vi "Get Path UI.vi"() -> ()   [LabVIEW 2016, in "LV-Data.PGSQL.lvclass"]
uses:
  LV-Data.PGSQL.lvclass
panel:
  out "path_to_selected_column":string="llab_038:d001(TEST_TABLE--new_stuff(hippos))"
  out "selected_table":string="TEST_TABLE"
  in  "columns_list":i32(listbox)=1
  in  "tables_list":i32(listbox)=34
  in  "STOP":bool
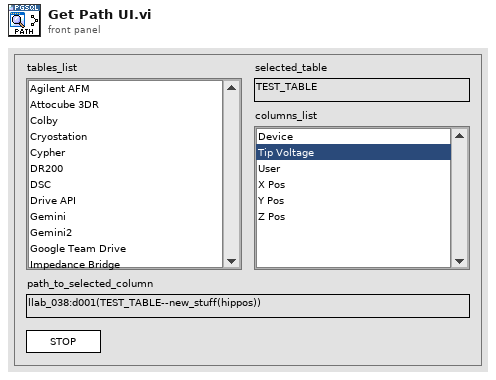
[diagram p1: front panel]
types:
  T1 = enum32{"Invalid", "Standard", "Closed", "Hidden", "Minimized", "Maximized"}
  T2 = enum32{"invalid app kind", "Development System", "Run Time System", "Student Edition", "Embedded LabVIEW", "Evaluation", "Custom"}
  T3 = cluster{"Core":cluster{"Current VI Reference":refnum<vi>, "Close Panel on Exit?":bool}, "Data.PG":refnum<class "LV-Data.PGSQL.lvclass">, "table names":string[], "table paths":string[], "column names":string[], "column units":string[], "column paths":string[], "new table name":string, "new column name":string, "new column data type":string, "new column units":string, "selected table":string, "selected column":string, "selected table path":string, "selected column path":string, "max points":i32, "selected column units":string}
  T4 = cluster{"Current VI Reference":refnum<vi>, "Close Panel on Exit?":bool}
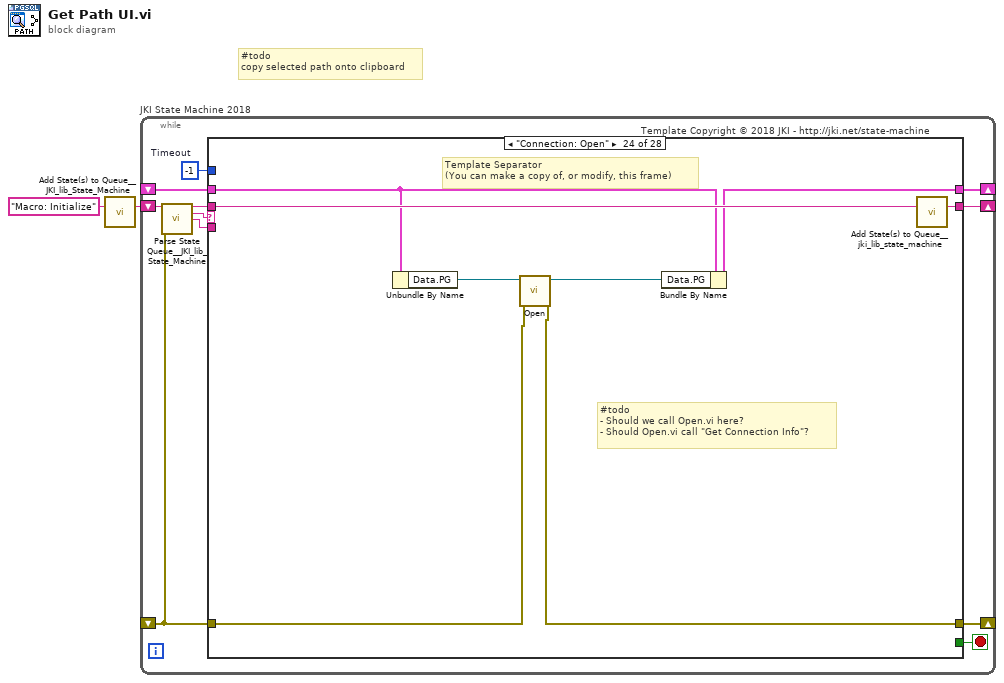
[diagram p0: block diagram]
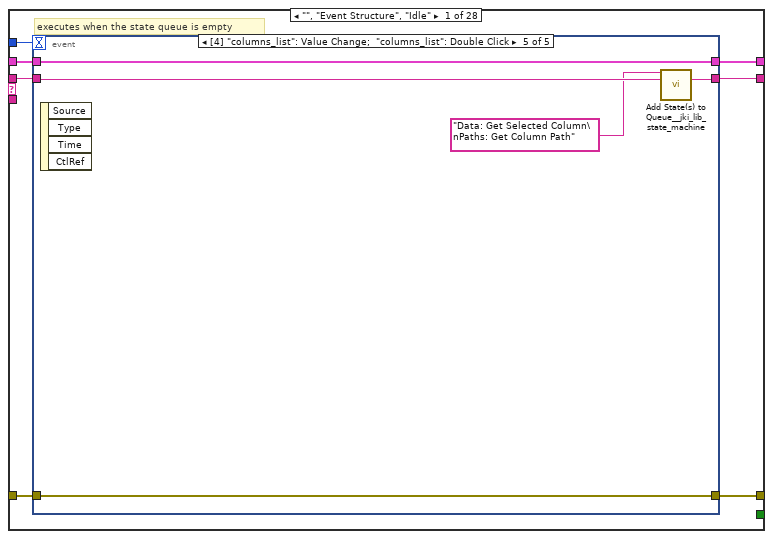
[diagram p2: hidden frame]
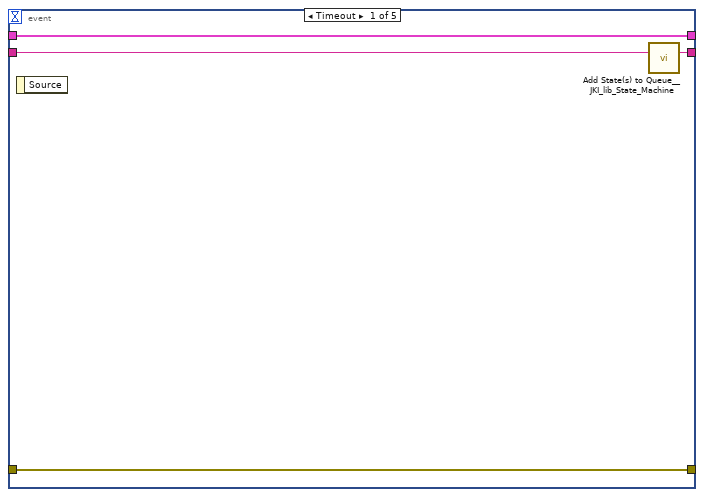
[diagram p3: hidden frame]
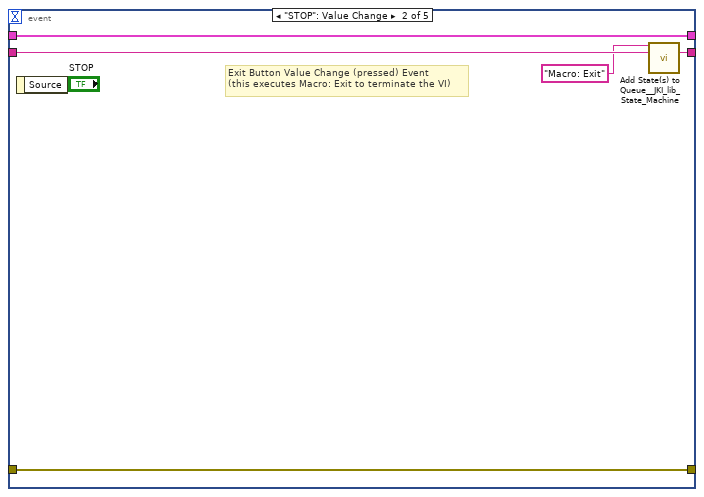
[diagram p4: hidden frame]
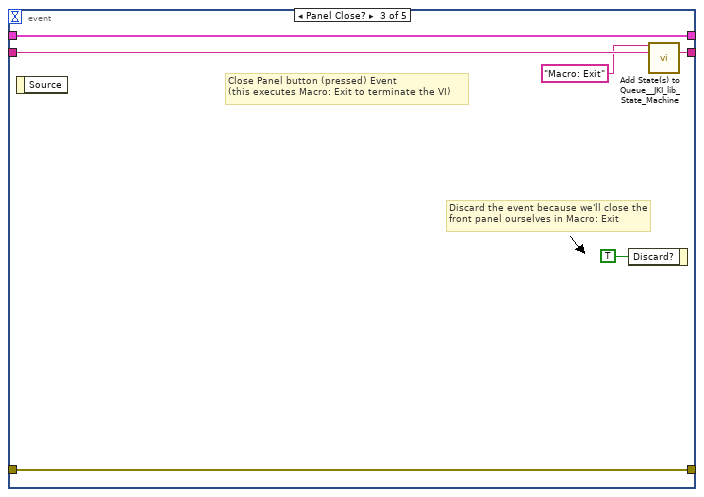
[diagram p5: hidden frame]
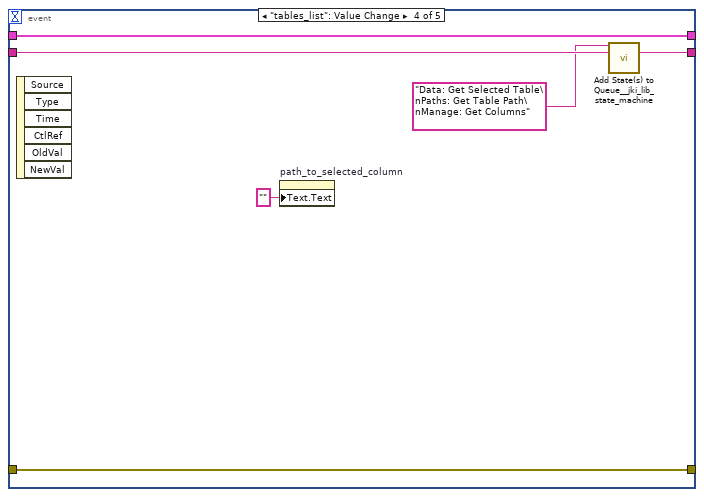
[diagram p6: hidden frame]
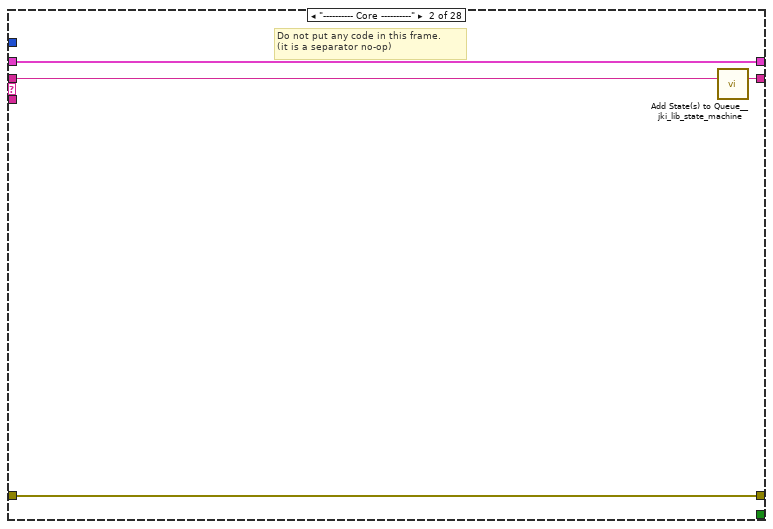
[diagram p7: hidden frame]
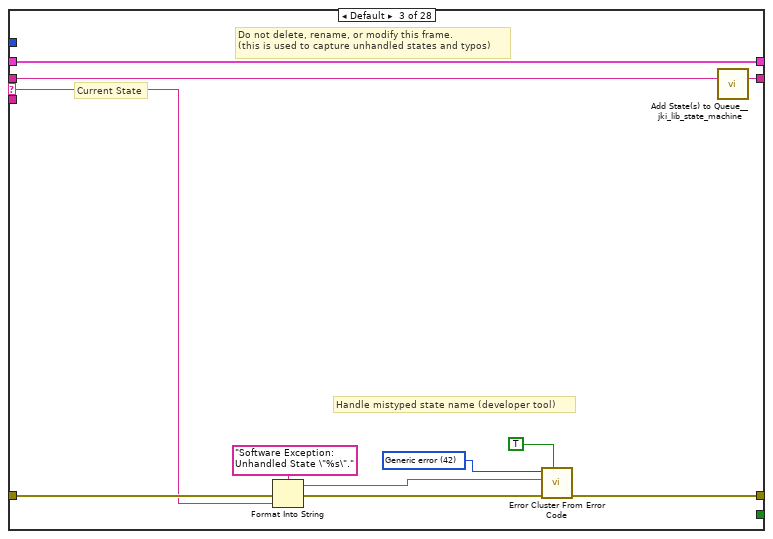
[diagram p8: hidden frame]
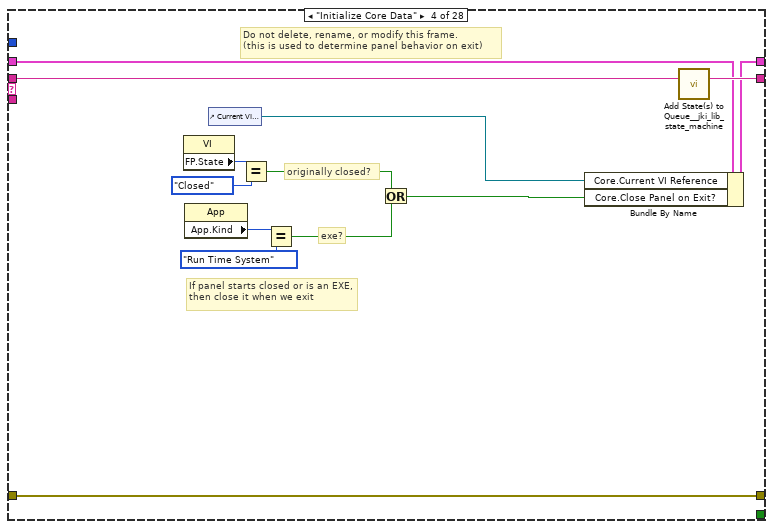
[diagram p9: hidden frame]
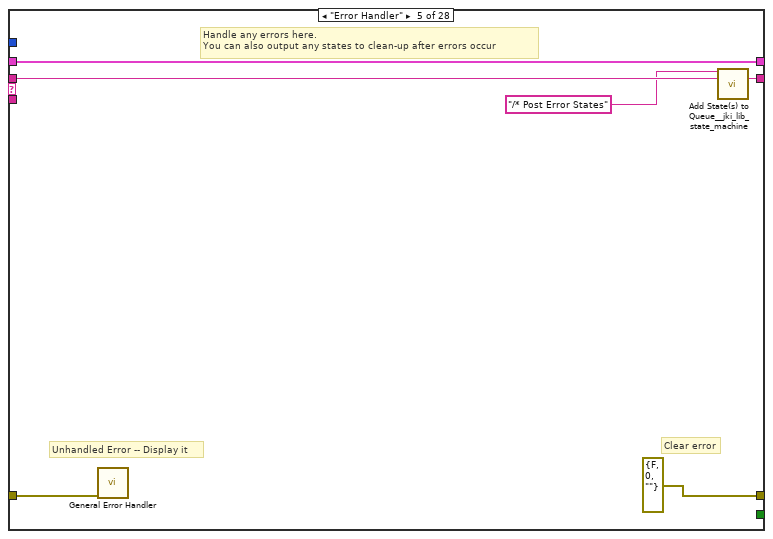
[diagram p10: hidden frame]
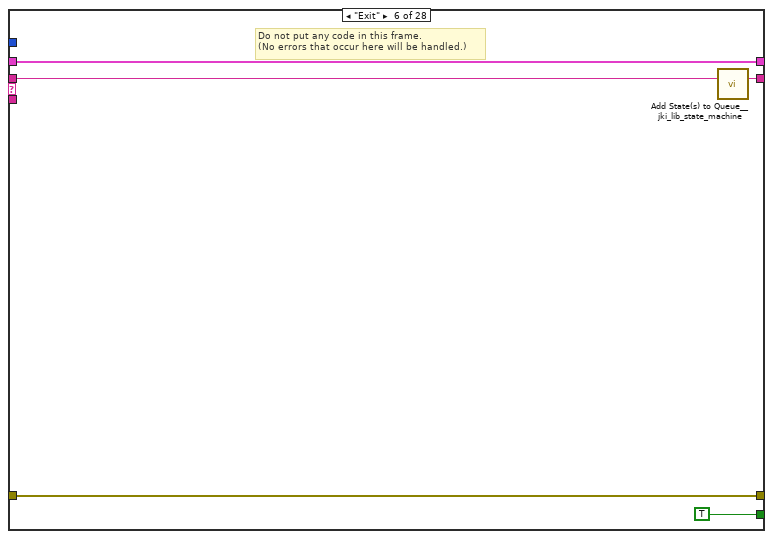
[diagram p11: hidden frame]
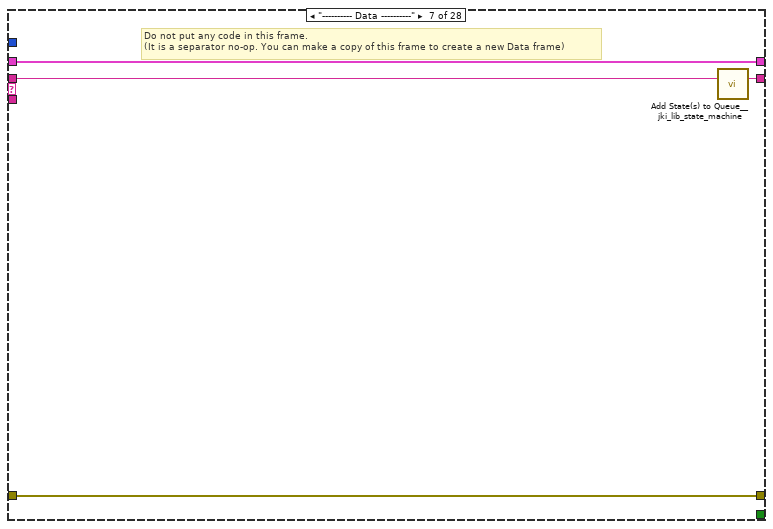
[diagram p12: hidden frame]
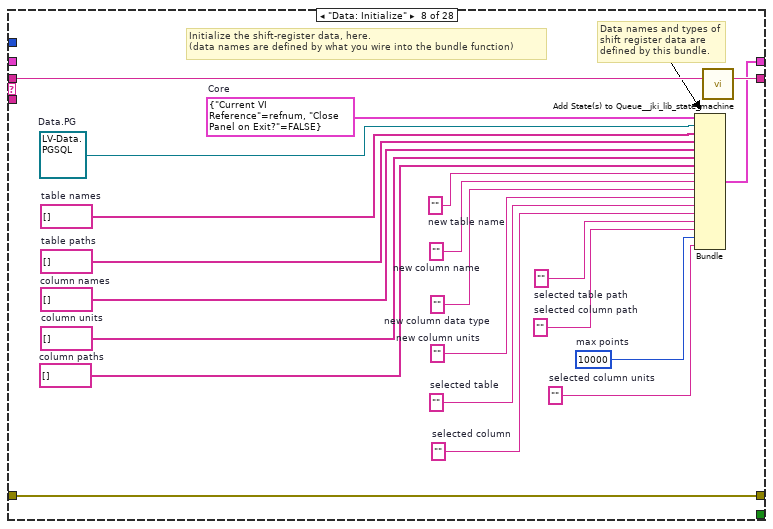
[diagram p13: hidden frame]
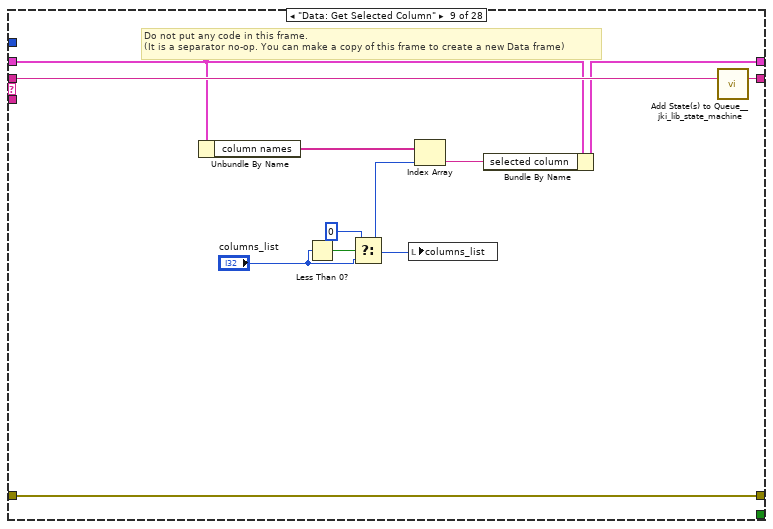
[diagram p14: hidden frame]
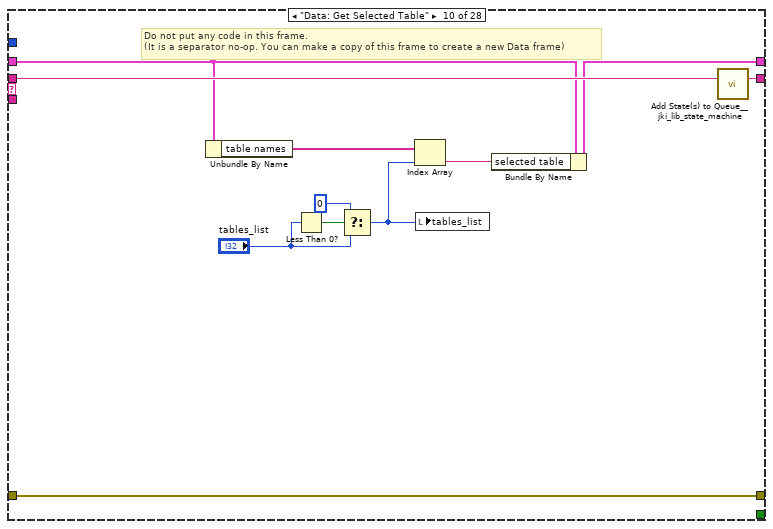
[diagram p15: hidden frame]
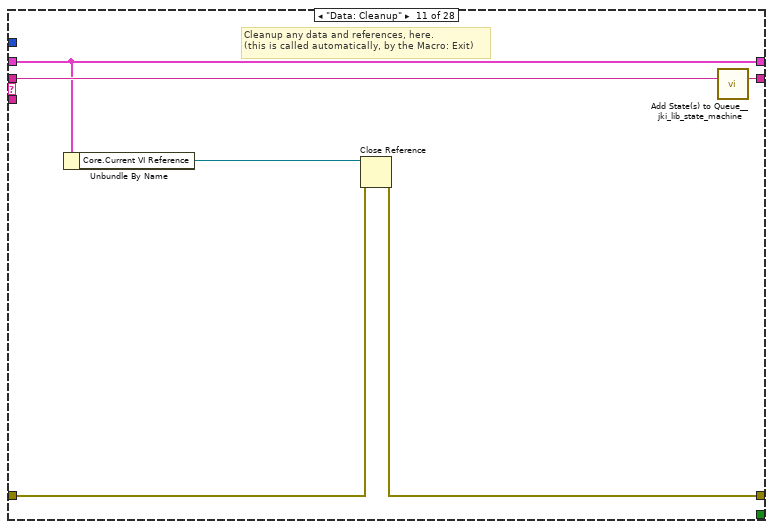
[diagram p16: hidden frame]
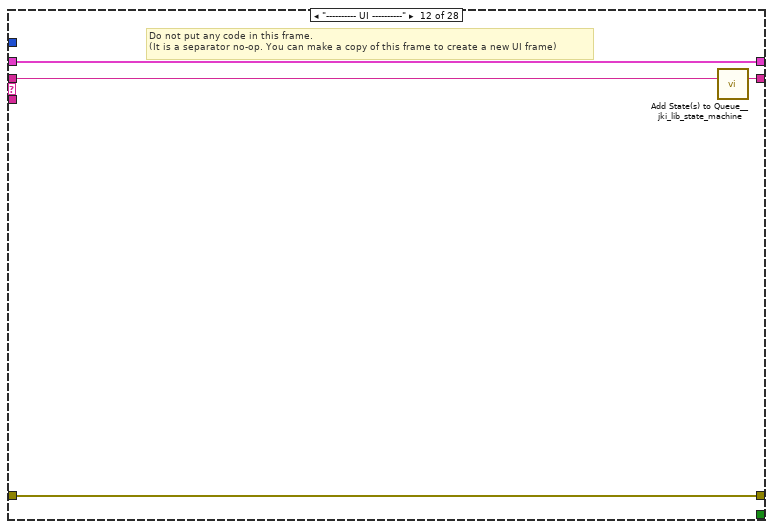
[diagram p17: hidden frame]
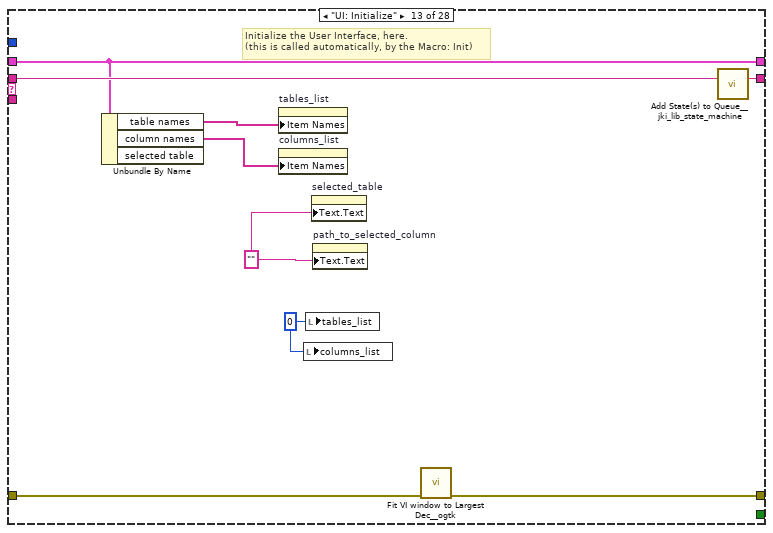
[diagram p18: hidden frame]
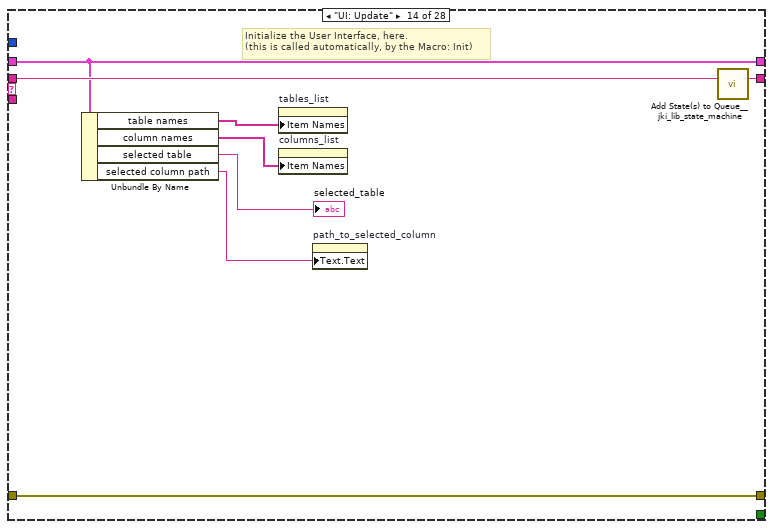
[diagram p19: hidden frame]
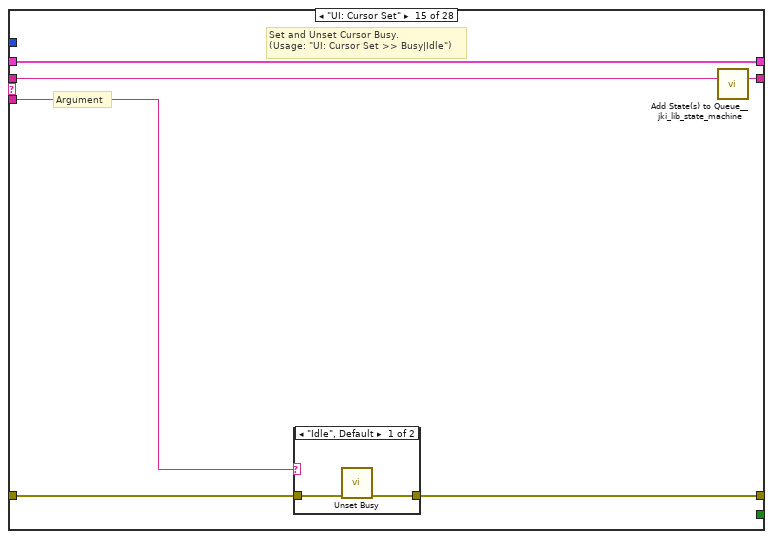
[diagram p20: hidden frame]
diagram:
  # "#todo\ncopy selected path onto clipboard"
  n1 = call <vilib>:"Add State(s) to Queue__JKI_lib_State_Machine.vi"("State(s) in (\"\")"="Macro: Initialize") -> ("States Out"=w2:string)  [unwired: 14 in]
  n2 = while "JKI State Machine 2018" {
    shift-right: [w6] -> _
    shift-left: _ -> [w5]
    shift-right: [w9] -> _
    shift-left: _ -> [w3]
    shift-right: [w8] -> _
    shift-left: w2 -> [w10]
    stop <- w7 stop-if-true
    w4 = -1  # Timeout
    # "Template Copyright © 2018 JKI - http://jki.net/state-machine"
    n3 = call <vilib>:"Parse State Queue__JKI_lib_State_Machine.vi"("State Queue"=w10, "Error In (no error)"=w3) -> ("Remaining States"=w12:string, "Current State"=w13:string, "Arguments"=w11:string)  [unwired: 11 in]
    n4 = case shown="\"Connection: Open\"" w13 {
      selector: w13 -> [_ _ w51 _ _ _ _ _ _ _ _ _ _ _ _ _ _ _ _ _ _ _ _ _ _ _ _ _]
      tunnel: w12 -> [w20 w50 w55 w74 w80 w85 w89 w110 w121 w132 w138 w142 w151 w159 w165 w176 w245 w250 w260 w264 w273 w286 w290 w298 w304 w308 w317 w331]
      tunnel: w11 -> [_ _ _ _ _ _ _ _ _ _ _ _ _ _ w160 w170 _ _ _ _ _ _ _ _ _ _ _ _]
      tunnel: w5 -> [w18 w47 w53 w67 w77 w83 w86 _ w116 w127 w134 w139 w147 w156 w163 w172 w242 w247 w257 w261 w269 w278 w287 w296 w302 w305 w313 w318]
      tunnel: [w17 w48 w57 w71 errorcluster {"status"=FALSE, "code"=0, "source"=""} ("error out") w82 w87 w107 w119 w130 w135 w140 w146 w155 w161 w173 w243 w248 w258 w262 w267 w280 w288 w292 w299 w306 w310 w326] -> w9
      tunnel: w3 -> [w16 w48 w56 w71 w76 w82 w87 w107 w119 w130 w133 w140 w145 w155 w162 w174 w243 w248 w258 w262 w268 w281 w288 w293 w300 w306 w311 w327]
      tunnel: [w19 w49 w54 w73 w79 w84 w88 w109 w120 w131 w137 w141 w150 w158 w164 w175 w244 w249 w259 w263 w272 w285 w289 w297 w303 w307 w316 w330] -> w8
      tunnel: [_ _ _ _ _ TRUE _ _ _ _ _ _ _ _ _ _ _ _ _ _ _ _ _ _ _ _ _ _] -> w7
      tunnel: [w15 w47 w53 w72 w77 w83 w86 w108 w115 w126 w134 w139 w147 w156 w163 w172 w242 w247 w257 w261 w270 w279 w287 w295 w302 w305 w309 w328] -> w6
      tunnel: w4 -> [w14 _ _ _ _ _ _ _ _ _ _ _ _ _ _ _ _ _ _ _ _ _ _ _ _ _ _ _]
      frame "", "Event Structure", "Idle" {
        # "executes when the state queue is empty"
        n5 = event shown="[4] \"columns_list\": Value Change;  \"columns_list\": Double Click" {
          selector: _ -> [_ _ _ _ _]
          dyn-events: _ -> [_ _ _ _ _]
          timeout: w14 -> [_ _ _ _ _]
          tunnel: w20 -> [w24 w29 w35 w39 w45]
          tunnel: [w23 w28 w34 w40 w46] -> w19
          tunnel: w18 -> [w21 w26 w32 w36 w42]
          tunnel: [w22 w27 w33 w41 w43] -> w17
          tunnel: w16 -> [w22 w27 w33 w41 w43]
          tunnel: [w21 w26 w32 w36 w42] -> w15
          event Timeout {
            n6 = event-data() -> ()  [unwired: 1 in, 1 out]
            n7 = call <vilib>:"Add State(s) to Queue__JKI_lib_State_Machine.vi"("State(s) in (\"\")"=w24) -> ("States Out"=w23:string)  [unwired: 14 in]
          }
          event "STOP": Value Change {
            # "Exit Button Value Change (pressed) Event\n(this executes Macro: Exit to terminate the VI)"
            n8 = event-data() -> ()  [unwired: 1 in, 1 out]
            n9 = call <vilib>:"Add State(s) to Queue__JKI_lib_State_Machine.vi"("State(s) in Front (\"\")"="Macro: Exit", "State(s) in (\"\")"=w29) -> ("States Out"=w28:string)  [unwired: 13 in]
          }
          event Panel Close? {
            # "Discard the event because we'll close the front panel ourselves in Macro: Exit"
            # "Close Panel button (pressed) Event\n(this executes Macro: Exit to terminate the VI)"
            n10 = event-data() -> ()  [unwired: 1 in, 1 out]
            n11 = event-data("Discard?"=TRUE) -> ()  [unwired: 1 in, 1 out]
            n12 = call <vilib>:"Add State(s) to Queue__JKI_lib_State_Machine.vi"("State(s) in Front (\"\")"="Macro: Exit", "State(s) in (\"\")"=w35) -> ("States Out"=w34:string)  [unwired: 13 in]
          }
          event "tables_list": Value Change {
            n13 = event-data() -> ()  [unwired: 1 in, 6 out]
            n14 = property on="path_to_selected_column" class="Str"("Text.Text"="") -> ()  [unwired: 2 in, 2 out]
            n15 = call <vilib>:"Add State(s) to Queue__jki_lib_state_machine.vi"("State(s) in Front (\"\")"="Data: Get Selected Table\nPaths: Get Table Path\nManage: Get Columns" ("State(s) in Front (\"\")"), "State(s) in (\"\")"=w39) -> ("States Out"=w40:string)  [unwired: 13 in]
          }
          event "columns_list": Value Change; "columns_list": Double Click {
            n16 = event-data() -> ()  [unwired: 1 in, 4 out]
            n17 = call <vilib>:"Add State(s) to Queue__jki_lib_state_machine.vi"("State(s) in Front (\"\")"="Data: Get Selected Column\nPaths: Get Column Path", "State(s) in (\"\")"=w45) -> ("States Out"=w46:string)  [unwired: 13 in]
          }
        }
      }
      frame "---------- Core ----------" {
        # "Do not put any code in this frame.\n(it is a separator no-op)"
        n18 = call <vilib>:"Add State(s) to Queue__jki_lib_state_machine.vi"("State(s) in (\"\")"=w50) -> ("States Out"=w49:string)  [unwired: 14 in]
      }
      frame Default {
        w60 = 42 items=["No error", "Argument error", "Memory is full", "Out of zone", "End of file", "File already open", "Generic file I/O error", "File not found", "File permission error", "Disk is full", "Duplicate path", "Too many files open", "System feature not enabled", "Resource file not found", "Cannot add resource", "Resource not found", "Image not found", "Image memory error", "Pen does not exist", "Config type invalid", "Config token not found", "Config parse error", "Config memory error", "Bad external code format", "Bad external code offset", "External code not present", "Null window", "Destroy window error", "Null menu", "Print aborted", "Bad print record", "Print driver error", "Windows error during printing", "Memory error during printing", "Print dialog error", "Generic print error", "Invalid device refnum", "Device not found", "Device parameter error", "Device unit error", "Cannot open device", "Device call aborted", "Generic error", "Cancelled by user", "Object ID too low", "Object ID too high", "Object not in heap", "Unknown heap", "Unknown object (invalid DefProc)", "Unknown object (DefProc not in table)", "Message out of range", "Invalid (null) method", "Unknown message", "Manager call not supported", "Bad address", "Network operation in progress", "Network operation timed out", "Connection is busy", "Network attribute not supported", "Network error", "Address in use", "System out of memory", "Connection aborted", "Connection refused", "Not connected", "Already connected", "Connection closed", "Initialization error (interapplication manager)", "Bad occurrence", "Wait on unbound occurrence handler", "Occurrence queue overflow", "Datalog type conflict", "Unused", "Unrecognized type (interapplication manager)", "Memory corrupt", "Failed to make temporary DLL", "Old CIN version", "Drag socket not found", "Failed to load drop-object", "Failed to register OLE object", "Failed to release OLE object", "Format specifier type mismatch", "Unknown format specifier", "Too few format specifiers", "Too many format specifiers", "Scan failed", "Newer CIN version", "Error converting to variant", "Runtime menu error", "Password tampered", "Variant attribute not found", "Incompatible variant data type", "Event data is not available", "Event Store is not present", "Occurrence is not found", "Event Queue is not created", "Event info is not available", "Refnum passed is NULL", "Error retrieving Class GUID", "Error retrieving CoClass GUID", "Error retrieving TypeLib GUID.", "Bad built application magic bytes.", "Specific driver is different from the specific driver associated with the Logical Name.", "There is no session opened to the class driver.", "Max Error", "MAX - Error with config objects", "MAX - Error loading configuration", "MAX - Group not supported"]
        # "Current State"
        # "Do not delete, rename, or modify this frame.\n(this is used to capture unhandled states and typos)"
        # "Handle mistyped state name (developer tool)"
        n19 = Format Into String(format string="Software Exception: Unhandled State \"%s\"." ("message"), error in=w56, w51) -> (resulting string=w59:string, error out=w58:errorcluster)  [unwired: 1 in]
        n20 = call <vilib>:"Error Cluster From Error Code.vi"("show call chain? (False)"=TRUE, "error in (no error)"=w58, "error message (\"\")"=w59, "error code (0)"=w60) -> ("error out"=w57:errorcluster)  [unwired: 5 in]
        n21 = call <vilib>:"Add State(s) to Queue__jki_lib_state_machine.vi"("State(s) in (\"\")"=w55) -> ("States Out"=w54:string)  [unwired: 14 in]
      }
      frame "Initialize Core Data" {
        # "Do not delete, rename, or modify this frame.\n(this is used to determine panel behavior on exit)"
        # "originally closed?"
        # "exe?"
        # "If panel starts closed or is an EXE, then close it when we exit"
        n22 = property class="VI"() -> ("FP.State"=w64:T1)  [unwired: 2 in, 2 out]
        n23 = property class="App"() -> ("App.Kind"=w70:T2)  [unwired: 2 in, 2 out]
        n24 = control-ref of="Current VI Reference"() -> (w65:refnum<vi>)
        n25 = Equal?(x=w64, y=T1."Closed" ("Front Panel Window:State")) -> (x = y?=w62:bool)
        n26 = Equal?(x=w70, y=T2."Run Time System" ("Application:Kind")) -> (x = y?=w68:bool)
        n27 = Or(x=w62, y=w68) -> (x .or. y?=w66:bool)
        n28 = Bundle By Name(cluster=w67, "Core.Current VI Reference"=w65, "Core.Close Panel on Exit?"=w66) -> (w72:T3)
        n29 = call <vilib>:"Add State(s) to Queue__jki_lib_state_machine.vi"("State(s) in (\"\")"=w74) -> ("States Out"=w73:string)  [unwired: 14 in]
      }
      frame "Error Handler" {
        # "Unhandled Error -- Display it"
        # "Handle any errors here.\nYou can also output any states to clean-up after errors occur"
        # "Clear error"
        n30 = call <vilib>:"General Error Handler.vi"("error in (no error)"=w76) -> ()  [unwired: 10 in, 5 out]
        n31 = call <vilib>:"Add State(s) to Queue__jki_lib_state_machine.vi"("State(s) in Front (\"\")"="/* Post Error States", "State(s) in (\"\")"=w80) -> ("States Out"=w79:string)  [unwired: 13 in]
      }
      frame "Exit" {
        # "Do not put any code in this frame.\n(No errors that occur here will be handled.)"
        n32 = call <vilib>:"Add State(s) to Queue__jki_lib_state_machine.vi"("State(s) in (\"\")"=w85) -> ("States Out"=w84:string)  [unwired: 14 in]
      }
      frame "---------- Data ----------" {
        # "Do not put any code in this frame.\n(It is a separator no-op. You can make a copy of this frame to create a new Data frame)"
        n33 = call <vilib>:"Add State(s) to Queue__jki_lib_state_machine.vi"("State(s) in (\"\")"=w89) -> ("States Out"=w88:string)  [unwired: 14 in]
      }
      frame "Data: Initialize" {
        w90 = ""  # selected column units
        w91 = 10000  # max points
        w92 = ""  # selected column path
        w93 = ""  # selected table path
        w94 = ""  # selected column
        w95 = ""  # selected table
        w96 = ""  # new column units
        w97 = ""  # new column data type
        w98 = ""  # new column name
        w99 = ""  # new table name
        w100 = string[] []  # column paths
        w101 = string[] []  # column units
        w102 = string[] []  # column names
        w103 = string[] []  # table paths
        w104 = string[] []  # table names
        w105 = refnum<class "LV-Data.PGSQL.lvclass"> refnum  # Data.PG
        w106 = T4 {"Current VI Reference"=refnum, "Close Panel on Exit?"=FALSE}  # Core
        # "Data names and types of shift register data are defined by this bundle."
        # "Initialize the shift-register data, here.\n(data names are defined by what you wire into the bundle function)"
        n34 = Bundle("Core"=w106, "Data.PG"=w105, "table names"=w104, "table paths"=w103, "column names"=w102, "column units"=w101, "column paths"=w100, "new table name"=w99, "new column name"=w98, "new column data type"=w97, "new column units"=w96, "selected table"=w95, "selected column"=w94, "selected table path"=w93, "selected column path"=w92, "max points"=w91, "selected column units"=w90) -> (w108:T3)  [unwired: 1 in]
        n35 = call <vilib>:"Add State(s) to Queue__jki_lib_state_machine.vi"("State(s) in (\"\")"=w110) -> ("States Out"=w109:string)  [unwired: 14 in]
      }
      frame "Data: Get Selected Column" {
        # "Do not put any code in this frame.\n(It is a separator no-op. You can make a copy of this frame to create a new Data frame)"
        n36 = Unbundle By Name(w116) -> ("column names"=w118:string[])
        n37 = Less Than 0?(x="columns_list") -> (x < 0?=w114:bool)
        n38 = Select(t=0, s=w114, f="columns_list") -> (s? t:f=w111:i32)
        n39 = local write "columns_list"(w111) -> ()
        n40 = Index Array(array=w118, index=w111) -> (element=w117:string)
        n41 = Bundle By Name(cluster=w116, "selected column"=w117) -> (w115:T3)
        n42 = call <vilib>:"Add State(s) to Queue__jki_lib_state_machine.vi"("State(s) in (\"\")"=w121) -> ("States Out"=w120:string)  [unwired: 14 in]
      }
      frame "Data: Get Selected Table" {
        # "Do not put any code in this frame.\n(It is a separator no-op. You can make a copy of this frame to create a new Data frame)"
        n43 = Unbundle By Name(w127) -> ("table names"=w129:string[])
        n44 = Less Than 0?(x="tables_list") -> (x < 0?=w125:bool)
        n45 = Select(t=0, s=w125, f="tables_list") -> (s? t:f=w123:i32)
        n46 = Index Array(array=w129, index=w123) -> (element=w128:string)
        n47 = local write "tables_list"(w123) -> ()
        n48 = Bundle By Name(cluster=w127, "selected table"=w128) -> (w126:T3)
        n49 = call <vilib>:"Add State(s) to Queue__jki_lib_state_machine.vi"("State(s) in (\"\")"=w132) -> ("States Out"=w131:string)  [unwired: 14 in]
      }
      frame "Data: Cleanup" {
        # "Cleanup any data and references, here.\n(this is called automatically, by the Macro: Exit)"
        n50 = Unbundle By Name(w134) -> ("Core.Current VI Reference"=w136:refnum<vi>)
        n51 = Close Reference(reference=w136, error in (no error)=w133) -> (error out=w135:errorcluster)
        n52 = call <vilib>:"Add State(s) to Queue__jki_lib_state_machine.vi"("State(s) in (\"\")"=w138) -> ("States Out"=w137:string)  [unwired: 14 in]
      }
      frame "---------- UI ----------" {
        # "Do not put any code in this frame.\n(It is a separator no-op. You can make a copy of this frame to create a new UI frame)"
        n53 = call <vilib>:"Add State(s) to Queue__jki_lib_state_machine.vi"("State(s) in (\"\")"=w142) -> ("States Out"=w141:string)  [unwired: 14 in]
      }
      frame "UI: Initialize" {
        w144 = 0 ("tables_list")
        w143 = "" ("Text.Text")
        # "Initialize the User Interface, here.\n(this is called automatically, by the Macro: Init)"
        n54 = Unbundle By Name(w147) -> ("table names"=w149:string[], "column names"=w148:string[])  [unwired: 1 out]
        n55 = property on="tables_list" class="LstBox (strict)"("Item Names"=w149) -> ()  [unwired: 2 in, 2 out]
        n56 = property on="columns_list" class="LstBox (strict)"("Item Names"=w148) -> ()  [unwired: 2 in, 2 out]
        n57 = local write "columns_list"(w144) -> ()
        n58 = local write "tables_list"(w144) -> ()
        n59 = property on="selected_table" class="Str"("Text.Text"=w143) -> ()  [unwired: 2 in, 2 out]
        n60 = property on="path_to_selected_column" class="Str"("Text.Text"=w143) -> ()  [unwired: 2 in, 2 out]
        n61 = call <userlib>:"Fit VI window to Largest Dec__ogtk.vi"("error in (no error)"=w145) -> ("error out"=w146:errorcluster)  [unwired: 5 in, 1 out]
        n62 = call <vilib>:"Add State(s) to Queue__jki_lib_state_machine.vi"("State(s) in (\"\")"=w151) -> ("States Out"=w150:string)  [unwired: 14 in]
      }
      frame "UI: Update" {
        # "Initialize the User Interface, here.\n(this is called automatically, by the Macro: Init)"
        n63 = Unbundle By Name(w156) -> ("table names"=w157:string[], "column names"=w153:string[], "selected table"=→"selected_table":string, "selected column path"=w152:string)
        n64 = property on="tables_list" class="LstBox (strict)"("Item Names"=w157) -> ()  [unwired: 2 in, 2 out]
        n65 = property on="columns_list" class="LstBox (strict)"("Item Names"=w153) -> ()  [unwired: 2 in, 2 out]
        n66 = property on="path_to_selected_column" class="Str"("Text.Text"=w152) -> ()  [unwired: 2 in, 2 out]
        n67 = call <vilib>:"Add State(s) to Queue__jki_lib_state_machine.vi"("State(s) in (\"\")"=w159) -> ("States Out"=w158:string)  [unwired: 14 in]
      }
      frame "UI: Cursor Set" {
        # "Argument"
        # "Set and Unset Cursor Busy.\n(Usage: \"UI: Cursor Set >> Busy|Idle\")"
        n68 = case shown="\"Idle\", Default" w160 {
          tunnel: w162 -> [w167 w169]
          tunnel: [w166 w168] -> w161
          frame "Idle", Default {
            n69 = call <vilib>:"Unset Busy.vi"("error in (no error)"=w167) -> ("error out"=w166:errorcluster)  [unwired: 10 in]
          }
          frame "Busy" {
            n70 = call <vilib>:"Set Busy.vi"("error in (no error)"=w169) -> ("error out"=w168:errorcluster)  [unwired: 9 in, 1 out]
          }
        }
        n71 = call <vilib>:"Add State(s) to Queue__jki_lib_state_machine.vi"("State(s) in (\"\")"=w165) -> ("States Out"=w164:string)  [unwired: 14 in]
      }
      frame "UI: Front Panel State" {
        # "Argument"
        # "Set Front Panel Open or Closed\n(Usage: \"UI: Front Panel State >> Open|Close\")"
        n72 = Unbundle By Name(w172) -> ("Core.Current VI Reference"=w171:refnum<vi>)
        n73 = case shown="\"Open\", \"Standard\", Default" w170 {
          tunnel: w174 -> [w182 w197 w208 w221 w234]
          tunnel: [w184 w198 w210 w223 w236] -> w173
          tunnel: w171 -> [w183 w195 w209 w222 w235]
          frame "Open", "Standard", Default {
            w177 = T1."Standard" ("State")
            n74 = property class="VI"(reference=w183, error in=w182) -> (reference out=w180:refnum<vi>, error out=w181:errorcluster, "FP.State"=w179:T1)
            n75 = Not Equal?(x=w179, y=w177) -> (x != y?=w178:bool)
            n76 = case shown="False" w178 {
              tunnel: [w188 w190] -> w184
              tunnel: w181 -> [w187 w190]
              tunnel: w180 -> [w186 _]
              tunnel: w177 -> [w185 _]
              frame True {
                n77 = invoke class="VI" method="FP.Open"(reference=w186, error in=w187, "Activate"=TRUE, "State"=w185) -> (error out=w188:errorcluster)  [unwired: 1 in, 4 out]
              }
              frame False {
              }
            }
          }
          frame "Close", "Closed" {
            n78 = property class="VI"(reference=w195, error in=w197) -> (reference out=w194:refnum<vi>, error out=w196:errorcluster, "FP.State"=w192:T1)
            n79 = Not Equal?(x=w192, y=T1."Closed" ("Front Panel Window:State")) -> (x != y?=w191:bool)
            n80 = case shown="True" w191 {
              tunnel: [w199 w202] -> w198
              tunnel: w196 -> [w199 w201]
              tunnel: w194 -> [_ w200]
              frame False {
              }
              frame True {
                n81 = invoke class="VI" method="FP.Close"(reference=w200, error in=w201) -> (error out=w202:errorcluster)  [unwired: 1 in, 2 out]
              }
            }
          }
          frame "Hidden", "Hide" {
            w203 = T1."Hidden" ("State")
            n82 = property class="VI"(reference=w209, error in=w208) -> (reference out=w206:refnum<vi>, error out=w207:errorcluster, "FP.State"=w205:T1)
            n83 = Not Equal?(x=w205, y=w203) -> (x != y?=w204:bool)
            n84 = case shown="True" w204 {
              tunnel: [w214 w215] -> w210
              tunnel: w207 -> [w213 w215]
              tunnel: w206 -> [w212 _]
              tunnel: w203 -> [w211 _]
              frame True {
                n85 = invoke class="VI" method="FP.Open"(reference=w212, error in=w213, "State"=w211) -> (error out=w214:errorcluster)  [unwired: 2 in, 4 out]
              }
              frame False {
              }
            }
          }
          frame "Minimize", "Minimized" {
            w216 = T1."Minimized" ("State")
            n86 = property class="VI"(reference=w222, error in=w221) -> (reference out=w219:refnum<vi>, error out=w220:errorcluster, "FP.State"=w218:T1)
            n87 = Not Equal?(x=w218, y=w216) -> (x != y?=w217:bool)
            n88 = case shown="True" w217 {
              tunnel: [w227 w228] -> w223
              tunnel: w220 -> [w226 w228]
              tunnel: w219 -> [w225 _]
              tunnel: w216 -> [w224 _]
              frame True {
                n89 = invoke class="VI" method="FP.Open"(reference=w225, error in=w226, "State"=w224) -> (error out=w227:errorcluster)  [unwired: 2 in, 4 out]
              }
              frame False {
              }
            }
          }
          frame "Maximize", "Maximized" {
            w229 = T1."Maximized" ("State")
            n90 = property class="VI"(reference=w235, error in=w234) -> (reference out=w232:refnum<vi>, error out=w233:errorcluster, "FP.State"=w231:T1)
            n91 = Not Equal?(x=w231, y=w229) -> (x != y?=w230:bool)
            n92 = case shown="True" w230 {
              tunnel: [w240 w241] -> w236
              tunnel: w233 -> [w239 w241]
              tunnel: w232 -> [w238 _]
              tunnel: w229 -> [w237 _]
              frame True {
                n93 = invoke class="VI" method="FP.Open"(reference=w238, error in=w239, "State"=w237) -> (error out=w240:errorcluster)  [unwired: 2 in, 4 out]
              }
              frame False {
              }
            }
          }
        }
        n94 = call <vilib>:"Add State(s) to Queue__jki_lib_state_machine.vi"("State(s) in (\"\")"=w176) -> ("States Out"=w175:string)  [unwired: 14 in]
      }
      frame "---------- Macro ----------" {
        # "Do not put any code in this frame.\n(It is a separator no-op. You can make a copy of this frame to create a new Macro frame)"
        n95 = call <vilib>:"Add State(s) to Queue__jki_lib_state_machine.vi"("State(s) in (\"\")"=w245) -> ("States Out"=w244:string)  [unwired: 14 in]
      }
      frame "Macro: Initialize" {
        # "Initialization Macro\n(This is called once, when the VI starts)"
        n96 = call <vilib>:"Add State(s) to Queue__jki_lib_state_machine.vi"("State(s) in Front (\"\")"="Data: Initialize\nInitialize Core Data\nUI: Initialize\nUI: Front Panel State >> Open\n\nConnection: Open\nManage: Get Tables\nUI: Update\n\nData: Get Selected Table\nPaths: Get Table Path\n\nManage: Get Columns\nUI: Update\nData: Get Selected Column\n\nPaths: Get Column Path", "State(s) in (\"\")"=w250) -> ("States Out"=w249:string)  [unwired: 13 in]
      }
      frame "Macro: Exit" {
        # "Exit Macro\n(This is called once, when the VI exits)"
        n97 = Unbundle By Name(w257) -> ("Core.Close Panel on Exit?"=w256:bool)
        n98 = Select(t="UI: Front Panel State >> Close", s=w256, f="") -> (s? t:f=w253:string)
        n99 = call <vilib>:"Add State(s) to Queue__jki_lib_state_machine.vi"("State(s) in (\"\")"=w253, "State(s) at Back (\"\")"="Connection: Close\nData: Cleanup\nExit") -> ("States Out"=w251:string)  [unwired: 13 in]
        n100 = call <vilib>:"Add State(s) to Queue__jki_lib_state_machine.vi"("State(s) in Front (\"\")"=w251, "State(s) in (\"\")"=w260) -> ("States Out"=w259:string)  [unwired: 13 in]
      }
      frame "---------- Manage ----------" {
        # "Template Separator\n(You can make a copy of, or modify, this frame)"
        n101 = call <vilib>:"Add State(s) to Queue__jki_lib_state_machine.vi"("State(s) in (\"\")"=w264) -> ("States Out"=w263:string)  [unwired: 14 in]
      }
      frame "Manage: Get Tables" {
        # "Your code here.\n(You can make a copy of, or modify, this frame)"
        n102 = Unbundle By Name(w269) -> ("Data.PG"=w271:refnum<class "LV-Data.PGSQL.lvclass">)
        n103 = call "Get Tables.vi"("error in (no error)"=w268, "Data.PG"=w271) -> ("error out"=w267:errorcluster, "Table Paths"=w265:string[], "Table Names"=w266:string[])  [unwired: 6 in, 1 out]
        n104 = Bundle By Name(cluster=w269, "table names"=w266, "table paths"=w265) -> (w270:T3)
        n105 = call <vilib>:"Add State(s) to Queue__jki_lib_state_machine.vi"("State(s) in (\"\")"=w273) -> ("States Out"=w272:string)  [unwired: 14 in]
      }
      frame "Manage: Get Columns" {
        # "Your code here.\n(You can make a copy of, or modify, this frame)"
        n106 = Unbundle By Name(w278) -> ("Data.PG"=w284:refnum<class "LV-Data.PGSQL.lvclass">, "selected table path"=w283:string)
        n107 = call "Get Columns.vi"("error in (no error)"=w281, "Table Path"=w283, "Data.PG"=w284) -> ("error out"=w280:errorcluster, "Column Paths"=w276:string[], "Column Names"=w277:string[], "Data.PG out"=w274:refnum<class "LV-Data.PGSQL.lvclass">, "Column Units"=w275:string[])  [unwired: 4 in]
        n108 = Bundle By Name(cluster=w278, "Data.PG"=w274, "column names"=w277, "column paths"=w276, "column units"=w275) -> (w279:T3)
        n109 = call <vilib>:"Add State(s) to Queue__jki_lib_state_machine.vi"("State(s) in Front (\"\")"="UI: Update" ("State(s) in Front (\"\")"), "State(s) in (\"\")"=w286) -> ("States Out"=w285:string)  [unwired: 13 in]
      }
      frame "---------- Connection ----------" {
        # "Template Separator\n(You can make a copy of, or modify, this frame)"
        n110 = call <vilib>:"Add State(s) to Queue__jki_lib_state_machine.vi"("State(s) in (\"\")"=w290) -> ("States Out"=w289:string)  [unwired: 14 in]
      }
      frame "Connection: Open" {
        # "#todo\n- Should we call Open.vi here?\n- Should Open.vi call \"Get Connection Info\"?"
        # "Template Separator\n(You can make a copy of, or modify, this frame)"
        n111 = Unbundle By Name(w296) -> ("Data.PG"=w294:refnum<class "LV-Data.PGSQL.lvclass">)
        n112 = call-dynamic "Open.vi"("error in (no error)"=w293, "Data.PG in"=w294) -> ("error out"=w292:errorcluster, "Data.PG out"=w291:refnum<class "LV-Data.PGSQL.lvclass">)  [unwired: 8 in]
        n113 = Bundle By Name(cluster=w296, "Data.PG"=w291) -> (w295:T3)
        n114 = call <vilib>:"Add State(s) to Queue__jki_lib_state_machine.vi"("State(s) in (\"\")"=w298) -> ("States Out"=w297:string)  [unwired: 14 in]
      }
      frame "Connection: Close" {
        # "Template Separator\n(You can make a copy of, or modify, this frame)"
        n115 = Unbundle By Name(w302) -> ("Data.PG"=w301:refnum<class "LV-Data.PGSQL.lvclass">)
        n116 = call-dynamic "Close.vi"("error in (no error)"=w300, "Data.PG in"=w301) -> ("error out"=w299:errorcluster)  [unwired: 8 in, 1 out]
        n117 = call <vilib>:"Add State(s) to Queue__jki_lib_state_machine.vi"("State(s) in (\"\")"=w304) -> ("States Out"=w303:string)  [unwired: 14 in]
      }
      frame "---------- Paths ----------" {
        # "Template Separator\n(You can make a copy of, or modify, this frame)"
        n118 = call <vilib>:"Add State(s) to Queue__jki_lib_state_machine.vi"("State(s) in (\"\")"=w308) -> ("States Out"=w307:string)  [unwired: 14 in]
      }
      frame "Paths: Get Table Path" {
        # "Template Separator\n(You can make a copy of, or modify, this frame)"
        n119 = Unbundle By Name(w313) -> ("Data.PG"=w315:refnum<class "LV-Data.PGSQL.lvclass">, "selected table"=w314:string)
        n120 = call "Get Table Path.vi"("error in (no error)"=w311, "Table Name"=w314, "Data.PG"=w315) -> ("error out"=w310:errorcluster, "Table Path"=w312:string)  [unwired: 5 in, 2 out]
        n121 = Bundle By Name(cluster=w313, "selected table path"=w312) -> (w309:T3)
        n122 = call <vilib>:"Add State(s) to Queue__jki_lib_state_machine.vi"("State(s) in (\"\")"=w317) -> ("States Out"=w316:string)  [unwired: 14 in]
      }
      frame "Paths: Get Column Path" {
        # "Template Separator\n(You can make a copy of, or modify, this frame)"
        n123 = Unbundle By Name(w318) -> ("Data.PG"=w329:refnum<class "LV-Data.PGSQL.lvclass">, "selected table path"=w324:string, "selected column"=w320:string, "selected table"=w321:string, "selected column"=w325:string)
        n124 = call "Get Column Path.vi"("error in (no error)"=w327, "Column Name"=w320, "Table path"=w324, "Data.PG in"=w329) -> ("error out"=w326:errorcluster, "Column Unit"=w323:string, "Column Path"=w322:string)  [unwired: 4 in, 1 out]
        n125 = call "Build Path.vi"("Table path"=w324, "Column path"=w322, "Table name"=w321, "Column name"=w325, "Column units"=w323) -> ("PG path"=w319:string)  [unwired: 10 in]
        "path_to_selected_column" <- w319
        n126 = Bundle By Name(cluster=w318, "selected column path"=w322, "selected column units"=w323) -> (w328:T3)
        n127 = invoke class="App" method="Clipboard.Write"("Param 0"=w319) -> ()  [unwired: 3 in, 4 out]
        n128 = call <vilib>:"Add State(s) to Queue__jki_lib_state_machine.vi"("State(s) in (\"\")"=w331) -> ("States Out"=w330:string)  [unwired: 14 in]
      }
    }
  }
